vi "Write OCP_Enable.vi"(8 "error in":errorcluster, 10 "OCP_Enable":bool, 11 "6032A in":refnum<class "6032A.lvclass">) -> (0 "error out":errorcluster, 3 "6032A out":refnum<class "6032A.lvclass">)   [LabVIEW 2019, in "6032A.lvlib" / "6032A.lvclass"]
uses:
  Library/6032A.lvclass
  builds/Instruments/PowerSupply.lvlibp/Library/PowerSupply.lvclass
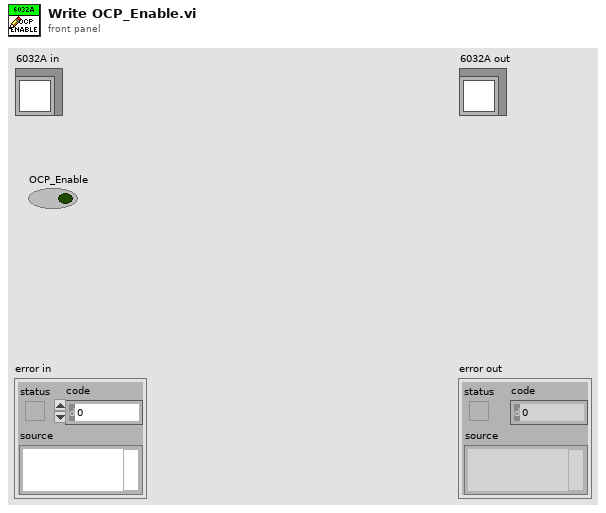
[diagram p1: front panel]
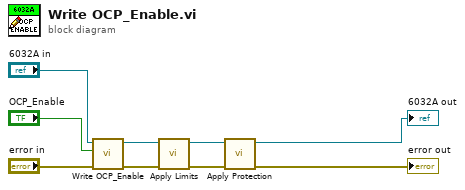
[diagram p0: block diagram]
diagram:
  n1 = call-parent "Write OCP_Enable.vi"("error in"="error in", "OCP_Enable"="OCP_Enable", "PowerSupply in"="6032A in") -> ("error out"=w5:errorcluster, "PowerSupply out"=w6:refnum<class "6032A.lvclass">)  [unwired: 7 in]
  n2 = call "Apply Limits.vi"("error in"=w5, "6032A in"=w6) -> ("error out"=w4:errorcluster, "6032A out"=w3:refnum<class "6032A.lvclass">)  [unwired: 8 in]
  n3 = call "Apply Protection.vi"("error in"=w4, "6032A in"=w3) -> ("error out"=→"error out":errorcluster, "6032A out"=→"6032A out":refnum<class "6032A.lvclass">)  [unwired: 8 in]
